vi "Pivot.vi"(9 "setpointValue":enum16{"90", "45", "0"}(ring), 10 "Output":dbl, 11 "Enum":enum16{"SetPoint", "Open", "Control"}(ring)) -> (2 "Distance":dbl)   [LabVIEW 2018]
uses:
  <vilib>/Rock Robotics/SystemInterfaces/DIO/FPGA_DIOChannel.ctl
  <vilib>/Rock Robotics/WPI/ThirdParty/Phoenix-LabVIEW/Motor Controller/Controls/CTRE_Phoenix_MotorControl_ControlMode.ctl
  <vilib>/Rock Robotics/WPI/Counter/WPI_CounterDigitalInputToDigitalSource.vi
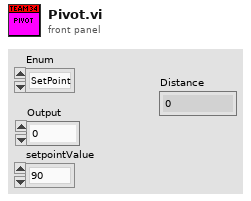
[diagram p1: front panel]
types:
  T1 = typedef "FPGA_DIOChannel.ctl" = enum8{"DIO 0", "DIO 1", "DIO 2", "DIO 3", "DIO 4", "DIO 5", "DIO 6", "DIO 7", "DIO 8", "DIO 9", "DIO MXP 0", "DIO MXP 1", "DIO MXP 2", "DIO MXP 3", "DIO MXP 4", "DIO MXP 5", "DIO MXP 6", "DIO MXP 7", "DIO MXP 8", "DIO MXP 9", "DIO MXP 10", "DIO MXP 11", "DIO MXP 12", "DIO MXP 13", "DIO MXP 14", "DIO MXP 15", "SPI Port CS1", "SPI Port CS2", "SPI Port CS3", "SPI Port MISO", "SPI Port MOSI", "Invalid"}
  T2 = typedef "WPI_MotorControlDeviceRef.ctl" = cluster{"DeviceStatus":errorcluster, "Type":T3, "PWM":cluster{"PWM Channel":T4, "DeadBand":T5}, "CAN":cluster{"Device Number":u8, "SetOutput VI Ref":variant, "GetOutput VI Ref":variant, "Enable VI Ref":variant, "Disable VI Ref":variant, "Data":variant}, "Invert":bool, "DIO PWM":cluster{"PWM \"Enable\" Channel":T4, "DIOChannel":T1, "PWM Rate":dbl}}
  T3 = typedef "WPI_MotorControlType.ctl" = enum16{"PWM", "CAN", "DIO PWM"}
  T4 = typedef "FPGA_DIOPWMChannel.ctl" = enum8{"PWM 0", "PWM 1", "PWM 2", "PWM 3", "PWM 4", "PWM 5", "PWM 6", "PWM 7", "PWM 8", "PWM 9", "PWM MXP 0", "PWM MXP 1", "PWM MXP 2", "PWM MXP 3", "PWM MXP 4", "PWM MXP 5", "PWM MXP 6", "PWM MXP 7", "PWM MXP 8", "PWM MXP 9", "Invalid"}
  T5 = typedef "WPI_PWMDeadband.ctl" = cluster{"Name":string, "maxPositivePwm":i32, "minPositivePwm":i32, "centerPwm":i32, "maxNegativePwm":i32, "minNegativePwm":i32, "angularRange":u16}
  T6 = typedef "WPI_DigitalInputDevRef.ctl" = cluster{"DevStatus":errorcluster, "DIO Channel":T1}
  T7 = typedef "FPGA_CounterEncoderSourceConvertionLVSourceType.ctl" = cluster{"DevStatus":errorcluster, "AnalogTriggerMode?":bool, "DigitalMode":cluster{"DIO Channel":T8}, "AnalogTriggerMode":cluster{"AnalogTriggerIndex":T9, "OutputType":T10}}
  T8 = typedef "FPGA_DIODigitalSourceChannel.ctl" = enum8{"DIO 0", "DIO 1", "DIO 2", "DIO 3", "DIO 4", "DIO 5", "DIO 6", "DIO 7", "DIO 8", "DIO 9", "DIO MXP 0", "DIO MXP 1", "DIO MXP 2", "DIO MXP 3", "DIO MXP 4", "DIO MXP 5", "DIO MXP 6", "DIO MXP 7", "DIO MXP 8", "DIO MXP 9", "DIO MXP 10", "DIO MXP 11", "DIO MXP 12", "DIO MXP 13", "DIO MXP 14", "DIO MXP 15", "SPI Port CS1", "SPI Port CS2", "SPI Port CS3", "SPI Port MISO", "SPI Port MOSI", "Disabled"}
  T9 = typedef "FPGA_AnalogTriggerIndex.ctl" = enum8{"Trig 0", "Trig 1", "Trig 2", "Trig 3", "Trig 4", "Trig 5", "Trig 6", "Trig 7", "Invalid"}
  T10 = typedef "FPGA_AnalogTriggerOutType.ctl" = enum16{"InWindow", "TriggerState", "Rising", "Falling"}
  T11 = typedef "WPI_EncoderDevRef.ctl" = cluster{"DevStatus":errorcluster, "EncoderIndex":T12, "CounterIndex":T13, "DistancePerCount":dbl, "Decoding Type":T14}
  T12 = typedef "FPGA_EncoderIdx.ctl" = enum8{"Enc 0", "Enc 1", "Enc 2", "Enc 3", "Enc 4", "Enc 5", "Enc 6", "Enc 7", "Invalid"}
  T13 = typedef "FPGA_CounterCtrSystemIndex.ctl" = enum8{"Ctr 0", "Ctr 1", "Ctr 2", "Ctr 3", "Ctr 4", "Ctr 5", "Ctr 6", "Ctr 7", "Invalid"}
  T14 = typedef "WPI_EncoderType.ctl" = enum16{"1x", "2x", "4x"}
  T15 = typedef "CTRE_Phoenix_MotorControl_ControlMode.ctl" = u16
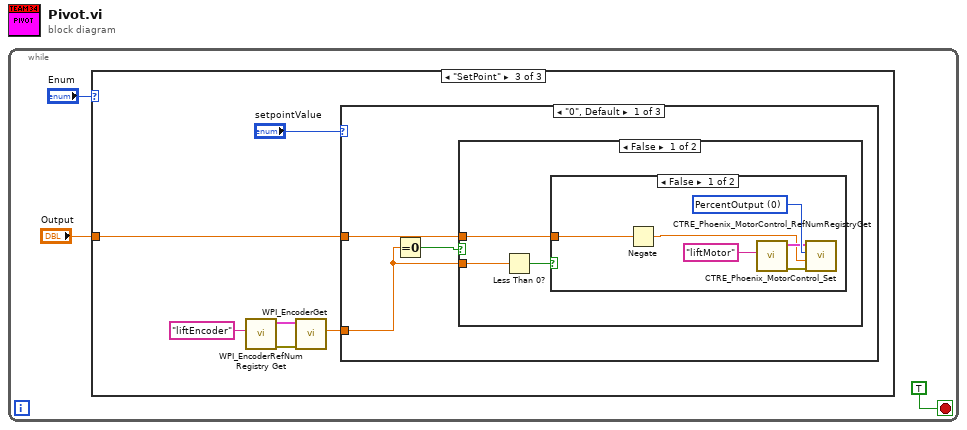
[diagram p0: block diagram]
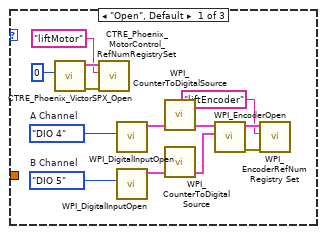
[diagram p2: hidden frame]
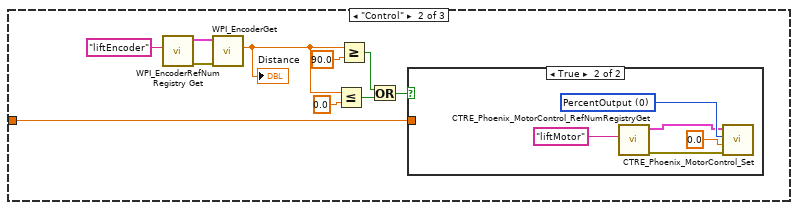
[diagram p3: hidden frame]
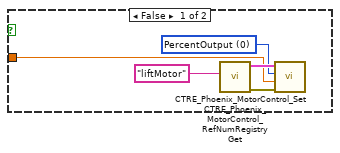
[diagram p4: hidden frame]
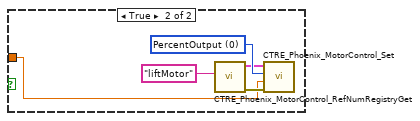
[diagram p5: hidden frame]
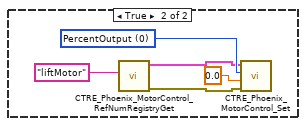
[diagram p6: hidden frame]
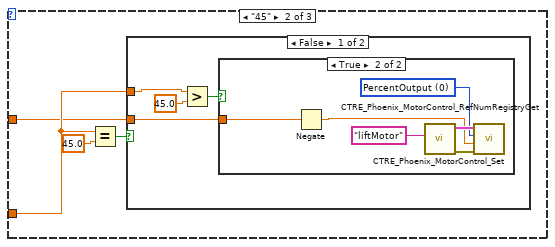
[diagram p7: hidden frame]
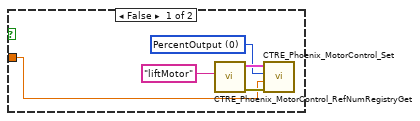
[diagram p8: hidden frame]
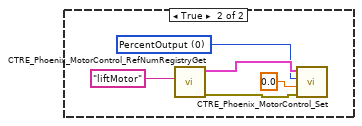
[diagram p9: hidden frame]
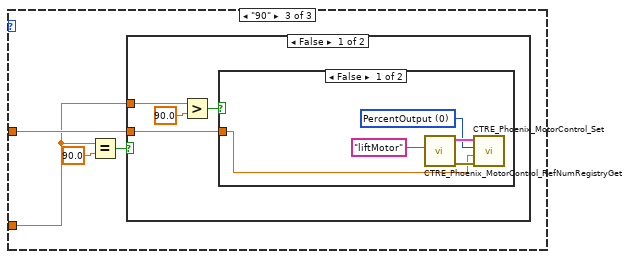
[diagram p10: hidden frame]
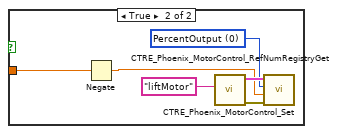
[diagram p11: hidden frame]
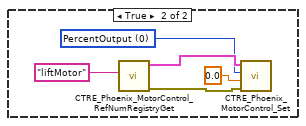
[diagram p12: hidden frame]
diagram:
  n1 = while {
    stop <- TRUE stop-if-true
    n2 = case shown="\"SetPoint\"" "Enum" {
      tunnel: "Output" -> [_ w17 w37]
      frame "Open", Default {
        w16 = FPGA_DIOChannel."DIO 5"  # B Channel
        w15 = FPGA_DIOChannel."DIO 4"  # A Channel
        n3 = call <vilib>:"CTRE_Phoenix_VictorSPX_Open.vi"("Device Number"=u8 0) -> ("error out"=w4:errorcluster, "CAN Talon SRX Ref"=w6:T2)  [unwired: 9 in]
        n4 = call <vilib>:"CTRE_Phoenix_MotorControl_RefNumRegistrySet.vi"("error in (no error)"=w4, "refnum name"="liftMotor", "PhoenixMotorControlDevRef"=w6) -> ()  [unwired: 7 in, 2 out]
        n5 = call <vilib>:"WPI_DigitalInputOpen.vi"("DIO Channel"=w15) -> ("DigitalInputDevRef"=w12:T6)  [unwired: 1 in, 9 out]
        n6 = call <vilib>:"WPI_DigitalInputOpen.vi"("DIO Channel"=w16) -> ("DigitalInputDevRef"=w13:T6)  [unwired: 1 in, 9 out]
        n7 = call-poly <vilib>:"WPI_CounterToDigitalSource.vi"("DigitalInputDevRef"=w12) -> ("Digital Source"=w11:T7)  [unwired: 6 out]
        n8 = call-poly <vilib>:"WPI_CounterToDigitalSource.vi"("DigitalInputDevRef"=w13) -> ("Digital Source"=w14:T7)  [unwired: 6 out]
        n9 = call <vilib>:"WPI_EncoderOpen.vi"("BSource"=w14, "ASource"=w11) -> ("error out"=w9:errorcluster, "EncoderDevRef"=w10:T11)  [unwired: 6 in, 2 out]
        n10 = call <vilib>:"WPI_EncoderRefNum Registry Set.vi"("error in (no error)"=w9, "refnum name"="liftEncoder", "EncoderDevRef"=w10) -> ()  [unwired: 7 in, 2 out]
      }
      frame "Control" {
        n11 = call <vilib>:"WPI_EncoderRefNum Registry Get.vi"("refnum name"="liftEncoder") -> ("error out"=w24:errorcluster, "EncoderDevRef"=w25:T11)  [unwired: 9 in]
        n12 = call <vilib>:"WPI_EncoderGet.vi"("error in (no error)"=w24, "EncoderDevRef"=w25) -> ("Distance"=w23:dbl)  [unwired: 4 in, 5 out]
        "Distance" <- w23
        n13 = Less Or Equal?(x=w23, y=0.0) -> (x <= y?=w22:bool)
        n14 = Greater Or Equal?(x=w23, y=90.0) -> (x >= y?=w21:bool)
        n15 = Or(x=w21, y=w22) -> (x .or. y?=w20:bool)
        n16 = case shown="True" w20 {
          tunnel: w17 -> [w27 _]
          frame False {
            w29 = T15 0 items=["PercentOutput"=0, "Position"=1, "Velocity"=2, "Current"=3, "Follower"=5, "MotionProfile"=6, "MotionMagic"=7, "MotionProfileArc"=10, "Disabled"=15] ("Control Mode")
            n17 = call <vilib>:"CTRE_Phoenix_MotorControl_RefNumRegistryGet.vi"("refnum name"="liftMotor") -> ("error out"=w31:errorcluster, "PhoenixMotorControlDevRef"=w30:T2)  [unwired: 9 in]
            n18 = call <vilib>:"CTRE_Phoenix_MotorControl_Set.vi"("error in (no error)"=w31, "Output"=w27, "Control Mode"=w29, "PhoenixMotorControlDevRef"=w30) -> ()  [unwired: 6 in, 2 out]
          }
          frame True {
            w36 = T15 0 items=["PercentOutput"=0, "Position"=1, "Velocity"=2, "Current"=3, "Follower"=5, "MotionProfile"=6, "MotionMagic"=7, "MotionProfileArc"=10, "Disabled"=15] ("Control Mode")
            n19 = call <vilib>:"CTRE_Phoenix_MotorControl_RefNumRegistryGet.vi"("refnum name"="liftMotor") -> ("error out"=w34:errorcluster, "PhoenixMotorControlDevRef"=w33:T2)  [unwired: 9 in]
            n20 = call <vilib>:"CTRE_Phoenix_MotorControl_Set.vi"("error in (no error)"=w34, "Output"=0.0 ("Output 2"), "Control Mode"=w36, "PhoenixMotorControlDevRef"=w33) -> ()  [unwired: 6 in, 2 out]
          }
        }
      }
      frame "SetPoint" {
        n21 = call <vilib>:"WPI_EncoderRefNum Registry Get.vi"("refnum name"="liftEncoder") -> ("error out"=w40:errorcluster, "EncoderDevRef"=w41:T11)  [unwired: 9 in]
        n22 = call <vilib>:"WPI_EncoderGet.vi"("error in (no error)"=w40, "EncoderDevRef"=w41) -> ("Distance"=w38:dbl)  [unwired: 4 in, 5 out]
        n23 = case shown="\"0\", Default" "setpointValue" {
          tunnel: w38 -> [w43 w66 w90]
          tunnel: w37 -> [w45 w65 w92]
          frame "0", Default {
            n24 = Equal To 0?(x=w43) -> (x = 0?=w44:bool)
            n25 = case shown="False" w44 {
              tunnel: w45 -> [w48 _]
              tunnel: w43 -> [w46 _]
              frame False {
                n26 = Less Than 0?(x=w46) -> (x < 0?=w47:bool)
                n27 = case shown="False" w47 {
                  tunnel: w48 -> [w50 w55]
                  frame False {
                    w54 = T15 0 items=["PercentOutput"=0, "Position"=1, "Velocity"=2, "Current"=3, "Follower"=5, "MotionProfile"=6, "MotionMagic"=7, "MotionProfileArc"=10, "Disabled"=15] ("Control Mode")
                    n28 = Negate(x=w50) -> (-x=w49:dbl)
                    n29 = call <vilib>:"CTRE_Phoenix_MotorControl_RefNumRegistryGet.vi"("refnum name"="liftMotor") -> ("error out"=w53:errorcluster, "PhoenixMotorControlDevRef"=w52:T2)  [unwired: 9 in]
                    n30 = call <vilib>:"CTRE_Phoenix_MotorControl_Set.vi"("error in (no error)"=w53, "Output"=w49, "Control Mode"=w54, "PhoenixMotorControlDevRef"=w52) -> ()  [unwired: 6 in, 2 out]
                  }
                  frame True {
                    w59 = T15 0 items=["PercentOutput"=0, "Position"=1, "Velocity"=2, "Current"=3, "Follower"=5, "MotionProfile"=6, "MotionMagic"=7, "MotionProfileArc"=10, "Disabled"=15] ("Control Mode")
                    n31 = call <vilib>:"CTRE_Phoenix_MotorControl_RefNumRegistryGet.vi"("refnum name"="liftMotor") -> ("error out"=w58:errorcluster, "PhoenixMotorControlDevRef"=w57:T2)  [unwired: 9 in]
                    n32 = call <vilib>:"CTRE_Phoenix_MotorControl_Set.vi"("error in (no error)"=w58, "Output"=w55, "Control Mode"=w59, "PhoenixMotorControlDevRef"=w57) -> ()  [unwired: 6 in, 2 out]
                  }
                }
              }
              frame True {
                w64 = T15 0 items=["PercentOutput"=0, "Position"=1, "Velocity"=2, "Current"=3, "Follower"=5, "MotionProfile"=6, "MotionMagic"=7, "MotionProfileArc"=10, "Disabled"=15] ("Control Mode")
                n33 = call <vilib>:"CTRE_Phoenix_MotorControl_RefNumRegistryGet.vi"("refnum name"="liftMotor") -> ("error out"=w63:errorcluster, "PhoenixMotorControlDevRef"=w62:T2)  [unwired: 9 in]
                n34 = call <vilib>:"CTRE_Phoenix_MotorControl_Set.vi"("error in (no error)"=w63, "Output"=0.0, "Control Mode"=w64, "PhoenixMotorControlDevRef"=w62) -> ()  [unwired: 6 in, 2 out]
              }
            }
          }
          frame "45" {
            n35 = Equal?(x=w66, y=45.0) -> (x = y?=w67:bool)
            n36 = case shown="False" w67 {
              tunnel: w66 -> [w72 _]
              tunnel: w65 -> [w70 _]
              frame False {
                n37 = Greater?(x=w72, y=45.0) -> (0:w69:bool)
                n38 = case shown="True" w69 {
                  tunnel: w70 -> [w73 w78]
                  frame False {
                    w74 = T15 0 items=["PercentOutput"=0, "Position"=1, "Velocity"=2, "Current"=3, "Follower"=5, "MotionProfile"=6, "MotionMagic"=7, "MotionProfileArc"=10, "Disabled"=15] ("Control Mode")
                    n39 = call <vilib>:"CTRE_Phoenix_MotorControl_RefNumRegistryGet.vi"("refnum name"="liftMotor") -> ("error out"=w75:errorcluster, "PhoenixMotorControlDevRef"=w76:T2)  [unwired: 9 in]
                    n40 = call <vilib>:"CTRE_Phoenix_MotorControl_Set.vi"("error in (no error)"=w75, "Output"=w73, "Control Mode"=w74, "PhoenixMotorControlDevRef"=w76) -> ()  [unwired: 6 in, 2 out]
                  }
                  frame True {
                    w80 = T15 0 items=["PercentOutput"=0, "Position"=1, "Velocity"=2, "Current"=3, "Follower"=5, "MotionProfile"=6, "MotionMagic"=7, "MotionProfileArc"=10, "Disabled"=15] ("Control Mode")
                    n41 = Negate(x=w78) -> (-x=w79:dbl)
                    n42 = call <vilib>:"CTRE_Phoenix_MotorControl_RefNumRegistryGet.vi"("refnum name"="liftMotor") -> ("error out"=w81:errorcluster, "PhoenixMotorControlDevRef"=w82:T2)  [unwired: 9 in]
                    n43 = call <vilib>:"CTRE_Phoenix_MotorControl_Set.vi"("error in (no error)"=w81, "Output"=w79, "Control Mode"=w80, "PhoenixMotorControlDevRef"=w82) -> ()  [unwired: 6 in, 2 out]
                  }
                }
              }
              frame True {
                w85 = T15 0 items=["PercentOutput"=0, "Position"=1, "Velocity"=2, "Current"=3, "Follower"=5, "MotionProfile"=6, "MotionMagic"=7, "MotionProfileArc"=10, "Disabled"=15] ("Control Mode")
                n44 = call <vilib>:"CTRE_Phoenix_MotorControl_RefNumRegistryGet.vi"("refnum name"="liftMotor") -> ("error out"=w86:errorcluster, "PhoenixMotorControlDevRef"=w87:T2)  [unwired: 9 in]
                n45 = call <vilib>:"CTRE_Phoenix_MotorControl_Set.vi"("error in (no error)"=w86, "Output"=0.0, "Control Mode"=w85, "PhoenixMotorControlDevRef"=w87) -> ()  [unwired: 6 in, 2 out]
              }
            }
          }
          frame "90" {
            n46 = Equal?(x=w90, y=90.0) -> (x = y?=w89:bool)
            n47 = case shown="False" w89 {
              tunnel: w90 -> [w96 _]
              tunnel: w92 -> [w94 _]
              frame False {
                n48 = Greater?(x=w96, y=90.0) -> (0:w93:bool)
                n49 = case shown="False" w93 {
                  tunnel: w94 -> [w97 w102]
                  frame False {
                    w98 = T15 0 items=["PercentOutput"=0, "Position"=1, "Velocity"=2, "Current"=3, "Follower"=5, "MotionProfile"=6, "MotionMagic"=7, "MotionProfileArc"=10, "Disabled"=15] ("Control Mode")
                    n50 = call <vilib>:"CTRE_Phoenix_MotorControl_RefNumRegistryGet.vi"("refnum name"="liftMotor") -> ("error out"=w99:errorcluster, "PhoenixMotorControlDevRef"=w100:T2)  [unwired: 9 in]
                    n51 = call <vilib>:"CTRE_Phoenix_MotorControl_Set.vi"("error in (no error)"=w99, "Output"=w97, "Control Mode"=w98, "PhoenixMotorControlDevRef"=w100) -> ()  [unwired: 6 in, 2 out]
                  }
                  frame True {
                    w104 = T15 0 items=["PercentOutput"=0, "Position"=1, "Velocity"=2, "Current"=3, "Follower"=5, "MotionProfile"=6, "MotionMagic"=7, "MotionProfileArc"=10, "Disabled"=15] ("Control Mode")
                    n52 = Negate(x=w102) -> (-x=w103:dbl)
                    n53 = call <vilib>:"CTRE_Phoenix_MotorControl_RefNumRegistryGet.vi"("refnum name"="liftMotor") -> ("error out"=w105:errorcluster, "PhoenixMotorControlDevRef"=w106:T2)  [unwired: 9 in]
                    n54 = call <vilib>:"CTRE_Phoenix_MotorControl_Set.vi"("error in (no error)"=w105, "Output"=w103, "Control Mode"=w104, "PhoenixMotorControlDevRef"=w106) -> ()  [unwired: 6 in, 2 out]
                  }
                }
              }
              frame True {
                w109 = T15 0 items=["PercentOutput"=0, "Position"=1, "Velocity"=2, "Current"=3, "Follower"=5, "MotionProfile"=6, "MotionMagic"=7, "MotionProfileArc"=10, "Disabled"=15] ("Control Mode")
                n55 = call <vilib>:"CTRE_Phoenix_MotorControl_RefNumRegistryGet.vi"("refnum name"="liftMotor") -> ("error out"=w110:errorcluster, "PhoenixMotorControlDevRef"=w111:T2)  [unwired: 9 in]
                n56 = call <vilib>:"CTRE_Phoenix_MotorControl_Set.vi"("error in (no error)"=w110, "Output"=0.0, "Control Mode"=w109, "PhoenixMotorControlDevRef"=w111) -> ()  [unwired: 6 in, 2 out]
              }
            }
          }
        }
      }
    }
  }
